vi "Open Session.vi"(8 "error in (no error)":errorcluster, 9 "replace if found? (F)":bool, 10 "create file if necessary (T)":bool=TRUE, 11 "configuration file path":path) -> (0 "error out":errorcluster, 1 "file replaced?":bool, 2 "file created?":bool, 3 "configuration session":refnum<class "Configuration Session.lvclass">, 4 "version":T1)   [LabVIEW 2020, in "DSF Core.lvlib" / "Configuration Session.lvclass"]
doc: "Opens a reference to the configuration data found in a platform-independent configuration file."
uses:
  Configuration Session.lvclass
  DSF Config Data.ctl
  Internal DSF Settings with ID.ctl
  Internal DSF Channel with ID.ctl
  Internal DSF Transfer with ID.ctl
  Typedefs/DSF Timing Info.ctl
  DSF Core.lvlib
  Internal DSF Group with ID.ctl
  Internal DSF Plugin with ID.ctl
  Typedefs/DSF Version Info.ctl
  Internal DSF Configuration.ctl
  Internal DSF Plugin Info.ctl
  Internal DSF Group Info.ctl
  Internal DSF Transfer Info.ctl
  Internal DSF Channel Info.ctl
  Internal DSF Settings Info.ctl
  Typedefs/DSF Settings Info.ctl
  Typedefs/DSF Engine Plugin Thread Configuration.ctl
  Typedefs/DSF Engine Framework Configuration.ctl
  Typedefs/DSF Engine Channel Configuration.ctl
  Typedefs/DSF Engine Transfer Configuration.ctl
  Typedefs/DSF Engine Transfer Group Configuration.ctl
  Typedefs/DSF Engine Plugin Configuration.ctl
  Typedefs/DSF Data Type.ctl
  Typedefs/Core Channel Configuration.ctl
  Configuration/Core/Channel/Channel Configuration.lvclass
  Typedefs/Core Transfer Configuration.ctl
  Configuration/Core/Transfer/Transfer Configuration.lvclass
  Typedefs/DSF Timeout Behavior.ctl
  Typedefs/DSF Direction.ctl
  Typedefs/Core Group Configuration.ctl
  Configuration/Core/Group/Group Configuration.lvclass
  Typedefs/Core Thread Configuration.ctl
  Configuration/Core/Thread/Thread Configuration.lvclass
  Typedefs/Core Plugin Configuration.ctl
  Configuration/Core/Plugin/Plugin Configuration.lvclass
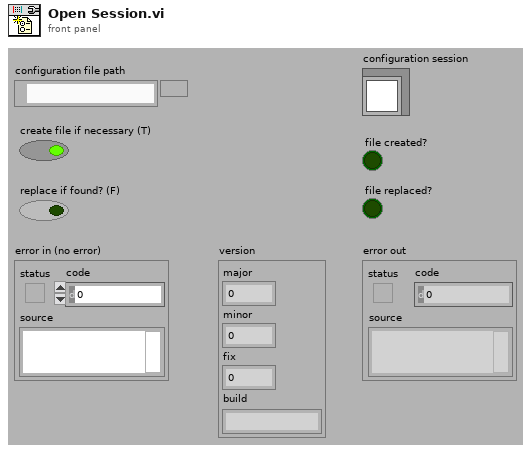
[diagram p1: front panel]
types:
  T1 = typedef "DSF Core.lvlib/DSF Version Info.ctl" = cluster{"major":u32, "minor":u32, "fix":u32, "build":string}
  T2 = typedef "DSF Core.lvlib/Configuration Session.lvclass/DSF Config Data.ctl" = cluster{"dsf configuration":T3, "path":path, "dirty":bool}
  T3 = typedef "DSF Core.lvlib/Configuration Session.lvclass/Internal DSF Configuration.ctl" = cluster{"dsfversion":T1, "version":T1, "plugins":T4[], "groups":T19[], "transfers":T21[], "channels":T23[], "settings":T25[], "framework configuration":T27, "configuration":refnum<class>}
  T4 = typedef "DSF Core.lvlib/Configuration Session.lvclass/Internal DSF Plugin with ID.ctl" = cluster{"id":string, "values":T5}
  T5 = typedef "DSF Core.lvlib/Configuration Session.lvclass/Internal DSF Plugin Info.ctl" = cluster{"components":string[], "timing":T6, "group ids":string[], "settings id":string, "threads":T7[]}
  T6 = typedef "DSF Core.lvlib/DSF Timing Info.ctl" = cluster{"priority":u64, "decimation":u64, "offset":u64}
  T7 = typedef "DSF Core.lvlib/DSF Engine Plugin Thread Configuration.ctl" = cluster{"core":T8, "component settings":T9[], "transfer groups":T10[]}
  T8 = typedef "DSF Core.lvlib/Thread Configuration.lvclass/Core Thread Configuration.ctl" = cluster{"processor":i32, "priority offset":i16}
  T9 = typedef "DSF Core.lvlib/DSF Settings Info.ctl" = cluster{"component":string, "values":cluster{"key":string, "value":string}[]}
  T10 = typedef "DSF Core.lvlib/DSF Engine Transfer Group Configuration.ctl" = cluster{"core":T11, "component settings":T9[], "transfers":T14[]}
  T11 = typedef "DSF Core.lvlib/Group Configuration.lvclass/Core Group Configuration.ctl" = cluster{"name":string, "direction":T12, "cycle timing":T6, "timeout behavior":T13, "enable conversion":bool}
  T12 = typedef "DSF Core.lvlib/DSF Direction.ctl" = enum8{"Tx", "Rx"}
  T13 = typedef "DSF Core.lvlib/DSF Timeout Behavior.ctl" = enum8{"Increment Late Count", "Throw Error"}
  T14 = typedef "DSF Core.lvlib/DSF Engine Transfer Configuration.ctl" = cluster{"core":T15, "component settings":T9[], "channels":T16[]}
  T15 = typedef "DSF Core.lvlib/Transfer Configuration.lvclass/Core Transfer Configuration.ctl" = cluster{"name":string}
  T16 = typedef "DSF Core.lvlib/DSF Engine Channel Configuration.ctl" = cluster{"core":T17, "component settings":T9[]}
  T17 = typedef "DSF Core.lvlib/Channel Configuration.lvclass/Core Channel Configuration.ctl" = cluster{"name":string, "units":string, "engine data type":T18, "string data type":T18, "string offset":u64}
  T18 = typedef "DSF Core.lvlib/DSF Data Type.ctl" = enum8{"Bool", "SGL", "DBL", "I8", "I16", "I32", "I64", "U8", "U16", "U32", "U64"}
  T19 = typedef "DSF Core.lvlib/Configuration Session.lvclass/Internal DSF Group with ID.ctl" = cluster{"id":string, "values":T20}
  T20 = typedef "DSF Core.lvlib/Configuration Session.lvclass/Internal DSF Group Info.ctl" = cluster{"direction":i32, "timing":T6, "transfer ids":string[], "settings id":string, "thread":i32, "timeout behavior":u8}
  T21 = typedef "DSF Core.lvlib/Configuration Session.lvclass/Internal DSF Transfer with ID.ctl" = cluster{"id":string, "values":T22}
  T22 = typedef "DSF Core.lvlib/Configuration Session.lvclass/Internal DSF Transfer Info.ctl" = cluster{"byte order":i32, "channel ids":string[], "settings id":string}
  T23 = typedef "DSF Core.lvlib/Configuration Session.lvclass/Internal DSF Channel with ID.ctl" = cluster{"id":string, "values":T24}
  T24 = typedef "DSF Core.lvlib/Configuration Session.lvclass/Internal DSF Channel Info.ctl" = cluster{"string buffer offset":u64, "string data type":i32, "engine data type":i32, "settings id":string, "units":string}
  T25 = typedef "DSF Core.lvlib/Configuration Session.lvclass/Internal DSF Settings with ID.ctl" = cluster{"id":string, "values":T26}
  T26 = typedef "DSF Core.lvlib/Configuration Session.lvclass/Internal DSF Settings Info.ctl" = cluster{"key":string, "value":string}[]
  T27 = typedef "DSF Core.lvlib/DSF Engine Framework Configuration.ctl" = cluster{"plugins":T28[]}
  T28 = typedef "DSF Core.lvlib/DSF Engine Plugin Configuration.ctl" = cluster{"core":T29, "component settings":T9[], "threads":T7[]}
  T29 = typedef "DSF Core.lvlib/Plugin Configuration.lvclass/Core Plugin Configuration.ctl" = cluster{"name":string, "components":string[], "cycle timing":T6}
  T30 = typedef "DSF Core.lvlib/Configuration Session.lvclass/DSF Config Data Ref.ctl" = refnum<data-value>
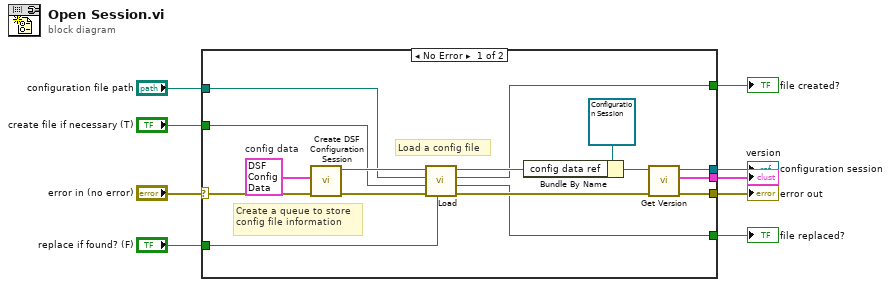
[diagram p0: block diagram]
diagram:
  n1 = case shown="No Error" "error in (no error)" {
    selector: "error in (no error)" -> [w25 w26]
    tunnel: "configuration file path" -> [w10 _]
    tunnel: "create file if necessary (T)" -> [w11 _]
    tunnel: [w13 _] -> w5
    tunnel: [w15 w26] -> w6
    tunnel: [w18 _] -> w4
    tunnel: "replace if found? (F)" -> [w23 _]
    tunnel: [w14 _] -> w2
    tunnel: [w16 _] -> w1
    frame No Error {
      w12 = T2 {"dsf configuration"={"dsfversion"={"major"=0, "minor"=0, "fix"=0, "build"=""}, "version"={"major"=0, "minor"=0, "fix"=0, "build"=""}, "plugins"=[], "groups"=[], "transfers"=[], "channels"=[], "settings"=[], "framework configuration"={"plugins"=[]}, "configuration"=refnum}, "path"=path "", "dirty"=FALSE}  # config data
      # "Load a config file"
      # "Create a queue to store config file information"
      n2 = call "Create DSF Configuration Session.vi"("error in (no error)"=w25, "config data"=w12) -> ("error out"=w24:errorcluster, "config data ref"=w22:T30)  [unwired: 8 in]
      n3 = call "Load.vi"("replace if found? (F)"=w23, "error in (no error)"=w24, "create file if necessary? (T)"=w11, "configuration file path"=w10, "config data ref in"=w22) -> ("error out"=w17:errorcluster, "file replaced?"=w14:bool, "file created?"=w13:bool, "config data ref out"=w20:T30)  [unwired: 3 out]
      n4 = Bundle By Name(cluster=refnum<class "Configuration Session.lvclass"> refnum ("Configuration Session in"), "config data ref"=w20) -> (w19:refnum<class "Configuration Session.lvclass">)
      n5 = call "Get Version.vi"("error in (no error)"=w17, "configuration session in"=w19) -> ("error out"=w15:errorcluster, "version"=w18:T1, "configuration session out"=w16:refnum<class "Configuration Session.lvclass">)  [unwired: 7 in]
    }
    frame Error {
    }
  }
  "error out" <- w6
  "file created?" <- w5
  "version" <- w4
  "file replaced?" <- w2
  "configuration session" <- w1
